vi "Index Counter.vi"(1 "Encoder Index (n-1)":i32, 2 "Change in Encoder Value":i32, 3 "Encoder Index Pin":bool, 4 "Encoder B Pin":bool, 5 "Encoder A Pin":bool, 6 "The Encoder Changed":bool) -> (0 "Encoder Index (n)":i32)   [LabVIEW 2010]
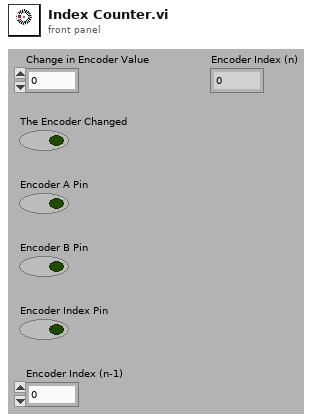
[diagram p1: front panel]
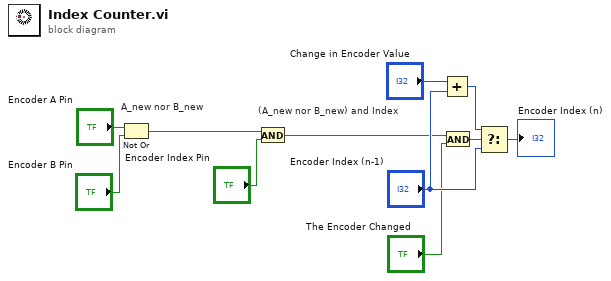
[diagram p0: block diagram]
diagram:
  n1 = Not Or "A_new nor B_new"(1:"Encoder B Pin", 2:"Encoder A Pin") -> (0:w3:bool)
  n2 = And "(A_new nor B_new) and Index"(x=w3, y="Encoder Index Pin") -> (x .and. y?=w10:bool)
  n3 = Add(x="Change in Encoder Value", y="Encoder Index (n-1)") -> (x+y=w8:i32)
  n4 = And(x=w10, y="The Encoder Changed") -> (x .and. y?=w6:bool)
  n5 = Select(t=w8, s=w6, f="Encoder Index (n-1)") -> (s? t:f=→"Encoder Index (n)":i32)
